vi "Timed One-Shot (SubVI).vi"(0 "ENABLE OUTPUT":bool, 7 "Time Setpoint [s]":dbl=10.0, 11 "START/RESET":bool) -> (4 "Output":bool, 8 "Elapsed Time [s]":dbl format="%.1f")   [LabVIEW 2012]
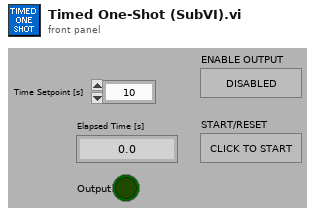
[diagram p1: front panel]
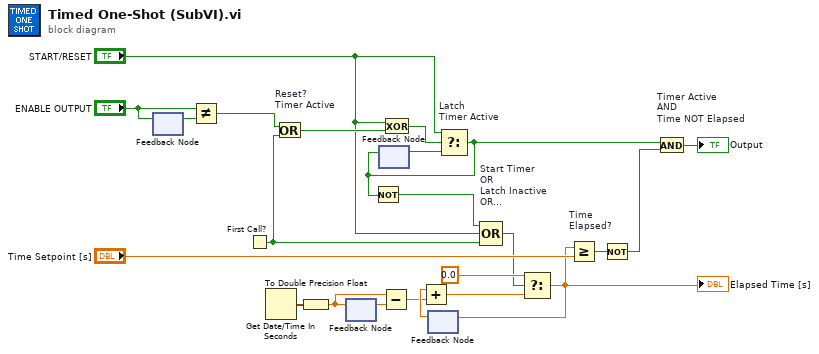
[diagram p0: block diagram]
diagram:
  n1 = feedback #1() -> (w19:bool)  [unwired: 1 in]
  n2 = feedback-in #1("ENABLE OUTPUT") -> ()
  n3 = Not Equal?(x="ENABLE OUTPUT", y=w19) -> (x != y?=w1:bool)
  n4 = First Call?() -> (First Call?: T/F=w8:bool)
  n5 = Get Date/Time In Seconds() -> (seconds since 1Jan1904=w15:timestamp)
  n6 = Or "Reset?\nTimer Active"(x=w1, y=w8) -> (x .or. y?=w22:bool)
  n7 = To Double Precision Float(number=w15) -> (double precision float=w14:dbl)
  n8 = feedback #2() -> (w16:dbl)  [unwired: 1 in]
  n9 = feedback-in #2(w14) -> ()
  n10 = feedback #3() -> (w21:bool)  [unwired: 1 in]
  n11 = Subtract(x=w14, y=w16) -> (x-y=w13:dbl)
  n12 = Exclusive Or(1:w22, 2:"START/RESET") -> (0:w20:bool)
  n13 = feedback #4() -> (w17:dbl)  [unwired: 1 in]
  n14 = Add(x=w17, y=w13) -> (x+y=w12:dbl)
  n15 = Select "Latch\nTimer Active"(t="START/RESET", s=w20, f=w21) -> (s? t:f=w6:bool)
  n16 = Not(x=w6) -> (.not. x?=w5:bool)
  n17 = feedback-in #3(w6) -> ()
  n18 = Compound Arithmetic op=OR "Start Timer\nOR\nLatch Inactive\nOR\nFirst Call"(w5, "START/RESET", w8) -> (w7:bool)
  n19 = Select(t=0.0, s=w7, f=w12) -> (s? t:f=w2:dbl)
  "Elapsed Time [s]" <- w2
  n20 = feedback-in #4(w2) -> ()
  n21 = Greater Or Equal? "Time\nElapsed?"(x=w2, y="Time Setpoint [s]") -> (x >= y?=w9:bool)
  n22 = Not(x=w9) -> (.not. x?=w10:bool)
  n23 = And "Timer Active\nAND\nTime NOT Elapsed"(x=w6, y=w10) -> (x .and. y?=→"Output":bool)
